vi "Write Sub Panel.vi"(8 "error in (no error)":errorcluster, 10 "Sub Panel":refnum<vi>, 11 "Mesage Display in":refnum<class "Mesage Display.lvclass">) -> (0 "error out":errorcluster, 3 "Mesage Display out":refnum<class "Mesage Display.lvclass">)   [LabVIEW 2020, in "Mesage Display.lvlib" / "Mesage Display.lvclass"]
uses:
  Mesage Display.lvclass
  Mesage Display.lvclass/Mesage Display.ctl
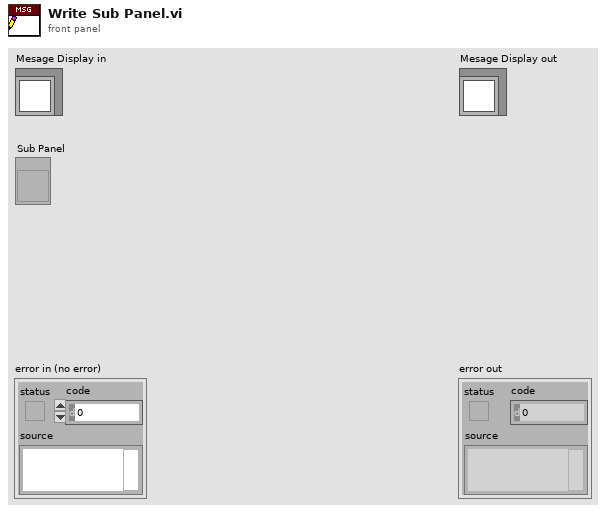
[diagram p1: front panel]
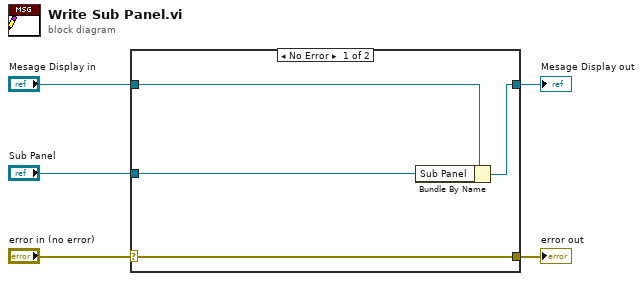
[diagram p0: block diagram]
diagram:
  n1 = case shown="No Error" "error in (no error)" {
    selector: "error in (no error)" -> [w9 w10]
    tunnel: [w9 w10] -> w4
    tunnel: [w7 w11] -> w2
    tunnel: "Mesage Display in" -> [w8 w11]
    tunnel: "Sub Panel" -> [w6 _]
    frame No Error {
      n2 = Bundle By Name(cluster=w8, "Sub Panel"=w6) -> (w7:refnum<class "Mesage Display.lvclass">)
    }
    frame Error {
    }
  }
  "error out" <- w4
  "Mesage Display out" <- w2
